vi "Send Email.vi"(5 "sComment":string, 6 "sSubject":string, 7 "sFrom":string, 8 "error in (no error)":errorcluster caption="错误输入（无错误）", 9 "sCC":string, 10 "sTo":string, 11 "Traceability 引用句柄":refnum<k24>) -> (0 "error out":errorcluster caption="错误输出", 2 "SendEmail":string, 3 "Traceability 引用句柄输出":refnum<k24>)   [LabVIEW 2014, in "Traceability.lvlib"]
uses:
  D:/webservice/Traceability.dll
  Traceability.dll
  Traceability.lvlib
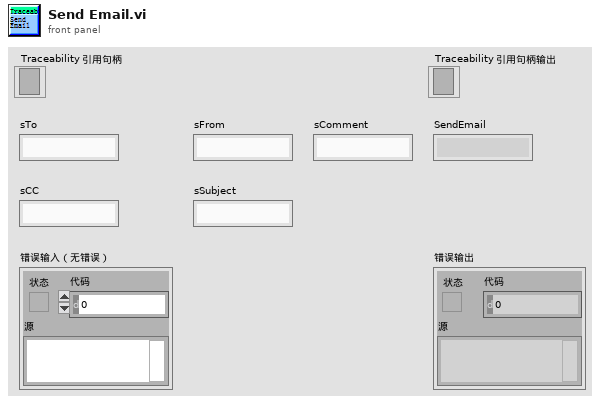
[diagram p1: front panel]
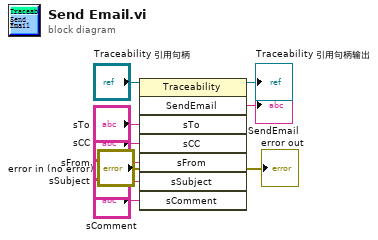
[diagram p0: block diagram]
diagram:
  n1 = invoke class="Traceability" method="SendEmail"(reference="Traceability 引用句柄", error in="error in (no error)", "sTo"="sTo", "sCC"="sCC", "sFrom"="sFrom", "sSubject"="sSubject", "sComment"="sComment") -> (reference out=→"Traceability 引用句柄输出":refnum<k24>, error out=→"error out":errorcluster, "SendEmail"=→"SendEmail":string)  [unwired: 1 in, 5 out]
